vi "WPI_IMU_ADIS16448_SPIDelay.vi"(8 "error in":errorcluster, 11 "SPIDevRef in":T1) -> (0 "error out":errorcluster, 3 "SPIDevRef out":T1)   [LabVIEW 2015, in "FRC ADI MXP IMU.lvlib"]
uses:
  FRC ADI MXP IMU.lvlib
  <vilib>/Rock Robotics/WPI/SPI/WPI_SPIDevRef.ctl
  <vilib>/Rock Robotics/SystemInterfaces/spilib/spi_bus.ctl
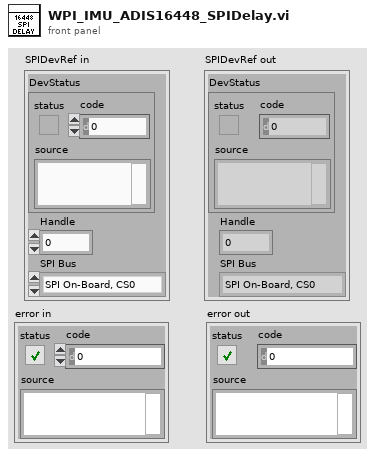
[diagram p1: front panel]
types:
  T1 = typedef "WPI_SPIDevRef.ctl" = cluster{"DevStatus":errorcluster, "Handle":i32, "SPI Bus":T2}
  T2 = typedef "spi_bus.ctl" = enum16{"SPI On-Board, CS0", "SPI On-Board, CS1", "SPI On-Board, CS2", "SPI On-Board, CS3", "SPI MXP", "Invalid"}
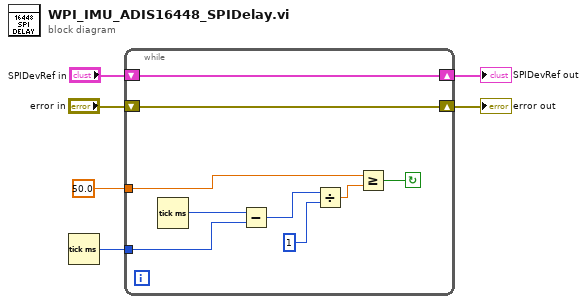
[diagram p0: block diagram]
diagram:
  n1 = Tick Count (ms)() -> (millisecond timer value=w5:u32)
  n2 = while {
    tunnel: 50.0 ("Delay (ms)") -> [w8]
    tunnel: w5 -> [w12]
    shift-right: [w15] -> w2
    shift-left: "error in" -> [w15]
    shift-right: [w14] -> w1
    shift-left: "SPIDevRef in" -> [w14]
    stop <- w7 continue-if-true
    n3 = Tick Count (ms)() -> (millisecond timer value=w13:u32)
    n4 = Subtract(x=w13, y=w12) -> (x-y=w11:u32)
    n5 = Divide(x=w11, y=u32 1) -> (x/y=w9:dbl)
    n6 = Greater Or Equal?(x=w8, y=w9) -> (x >= y?=w7:bool)
  }
  "SPIDevRef out" <- w1
  "error out" <- w2
